vi "Analyze Measurement Data.vi"(9 "measurementData":u32[](array[numeric]), 10 "outTarget":T1 items=["OUT01"=1, "OUT02"=2, "OUT03"=4, "OUT04"=8, "OUT05"=16, "OUT06"=32, "OUT07"=64, "OUT08"=128, "ALL OUT"=255], 11 "obtainedDataCount":u32) -> (3 "MEASUREMENT_DATA":T2[](array[typedef]) {"outMeasurementData"."judgeResult" items=["HI"=1, "GO"=2, "LO"=4]})   [LabVIEW 2020, in "Keyence CL-3000.lvlib"]
uses:
  Keyence CL-3000.lvlib
  Public/clusters/CL3IF_MEASUREMENT_DATA.ctl
  Public/clusters/CL3IF_OUTMEASUREMENT_DATA.ctl
  Public/enums/CL3IF_VALUE_INFO.ctl
  Public/enums/CL3IF_JUDGE_RESULT.ctl
  Public/enums/CL3IF_OUTNO.ctl
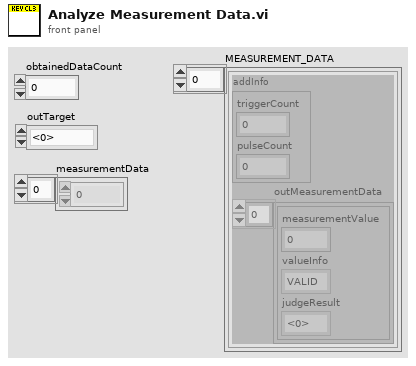
[diagram p1: front panel]
types:
  T1 = typedef "Keyence CL-3000.lvlib/CL3IF_OUTNO.ctl" = u16
  T2 = typedef "Keyence CL-3000.lvlib/CL3IF_MEASUREMENT_DATA.ctl" = cluster{"addInfo":cluster{"triggerCount":u32, "pulseCount":i32}, "outMeasurementData":T3[]}
  T3 = typedef "Keyence CL-3000.lvlib/CL3IF_OUTMEASUREMENT_DATA.ctl" = cluster{"measurementValue":i32, "valueInfo":T4, "judgeResult":T5}
  T4 = typedef "Keyence CL-3000.lvlib/CL3IF_VALUE_INFO.ctl" = enum8{"VALID", "JUDGMENTSTANDBY", "INVALID", "OVERDISPRANGE_P", "OVERDISPRANGE_N"}
  T5 = typedef "Keyence CL-3000.lvlib/CL3IF_JUDGE_RESULT.ctl" = u8
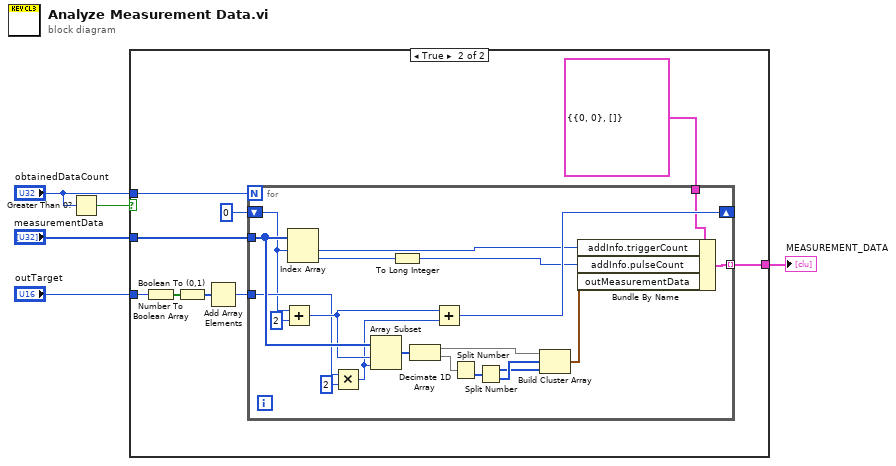
[diagram p0: block diagram]
diagram:
  n1 = Greater Than 0?(x="obtainedDataCount") -> (x > 0?=w1:bool)
  n2 = case shown="True" w1 {
    tunnel: [_ w6] -> w5
    tunnel: "measurementData" -> [_ w14]
    tunnel: "obtainedDataCount" -> [_ w13]
    tunnel: "outTarget" -> [_ w9]
    frame False {
    }
    frame True {
      n3 = Number To Boolean Array(number=w9) -> (Boolean array=w10:bool[])
      n4 = Boolean To (0,1)(Boolean=w10) -> (0, 1=w11:i16[])
      n5 = Add Array Elements(numeric array=w11) -> (sum=w8:i16)
      n6 = for {
        N: w13 -> [_]
        tunnel: w14 -> [w34]
        shift-right: [w30] -> _
        shift-left: 0 -> [w31]
        tunnel: w8 -> [w32]
        tunnel: T2 {"addInfo"={"triggerCount"=0, "pulseCount"=0}, "outMeasurementData"=[]} ("MEASUREMENT_DATA 2") -> [w24]
        tunnel: [w23] -> w6 mode=indexing
        n7 = Add(x=w31, y=2 ("x")) -> (x+y=w33:i32)
        n8 = Index Array(array=w34, index #1=w31) -> (element #1=w21:u32, element #2=w29:u32)  [unwired: 1 in]
        n9 = Multiply(x=w32, y=2) -> (x*y=w15:i32)
        n10 = Array Subset(array=w34, index=w33, length=w15) -> (w18:u32[])
        n11 = To Long Integer(number=w29) -> (32bit integer=w22:i32)
        n12 = Decimate 1D Array ("デシメート1D配列")(w18) -> (w27:u32[], w17:u32[])
        n13 = Add(x=w33, y=w15) -> (x+y=w30:i32)
        n14 = Split Number(x=w17) -> (lo(x)=w16:u16[])  [unwired: 1 out]
        n15 = Split Number(x=w16) -> (hi(x)=w25:u8[], lo(x)=w26:u8[])
        n16 = Build Cluster Array(w27, w26, w25) -> (w20:cluster{u32, u8, u8}[])
        n17 = Bundle By Name(cluster=w24, "addInfo.triggerCount"=w21, "addInfo.pulseCount"=w22, "outMeasurementData"=w20) -> (w23:T2)
      }
    }
  }
  "MEASUREMENT_DATA" <- w5
